vi "steerer range.vi"(4 "Steerer Y Voltage":dbl, 5 "Steerer X Voltage":dbl, 6 "Steerer Set Y":dbl, 7 "Steerer X Set":dbl) -> (3 "Steerer within range":bool)   [LabVIEW 2016, in "Low energy.lvlib"]
doc: "This vi takes the set valve from a X and Y steerer and subtracts the readbacks from the same steerer set. \nIt then compares to see if the power supplies are in within certain range."
uses:
  Low energy.lvlib
panel:
  out "Y Steerer Range":bool
  out "X Steerer Range":bool
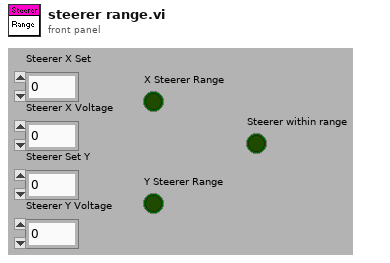
[diagram p1: front panel]
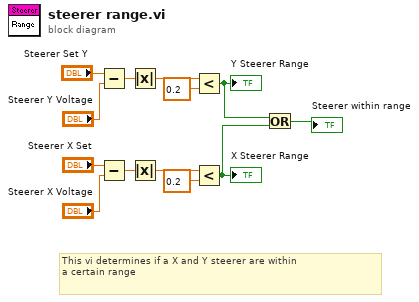
[diagram p0: block diagram]
diagram:
  # "This vi determines if a X and Y steerer are within\na certain range"
  n1 = Subtract(x="Steerer Set Y", y="Steerer Y Voltage") -> (x-y=w7:dbl)
  n2 = Subtract(x="Steerer X Set", y="Steerer X Voltage") -> (x-y=w12:dbl)
  n3 = Absolute Value(x=w7) -> (abs(x)=w6:dbl)
  n4 = Absolute Value(x=w12) -> (abs(x)=w13:dbl)
  n5 = Less?(x=w6, y=0.2) -> (x < y?=w3:bool)
  "Y Steerer Range" <- w3
  n6 = Less?(x=w13, y=0.2) -> (x < y?=w2:bool)
  "X Steerer Range" <- w2
  n7 = Or(x=w3, y=w2) -> (x .or. y?=→"Steerer within range":bool)
